vi "Gaussian surface graph.vi"(5 "output cluster":T1, 9 "plot number (1)":i32=2, 10 "X":dbl[](array[numeric]), 11 "Y":dbl[](array[numeric])) -> (0 "error out":errorcluster)   [LabVIEW 2023]
doc: "Generate Gaussian surface graph."
uses:
  <vilib>/Native 3D Graph/xcontrol/3DPC_SurfacePlot.xctl
  <vilib>/Native 3D Graph/classes/Base Datatype.lvclass
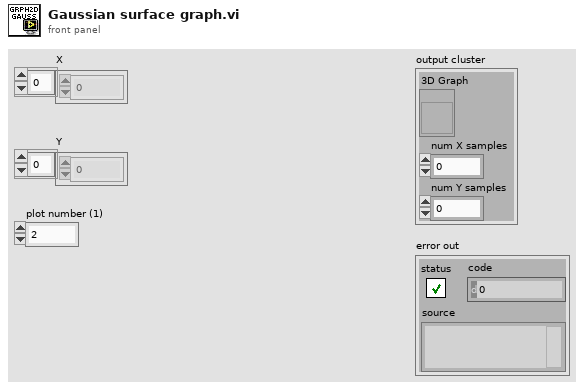
[diagram p1: front panel]
types:
  T1 = cluster{"3D Graph":refnum<vi>, "num X samples":i32, "num Y samples":i32}
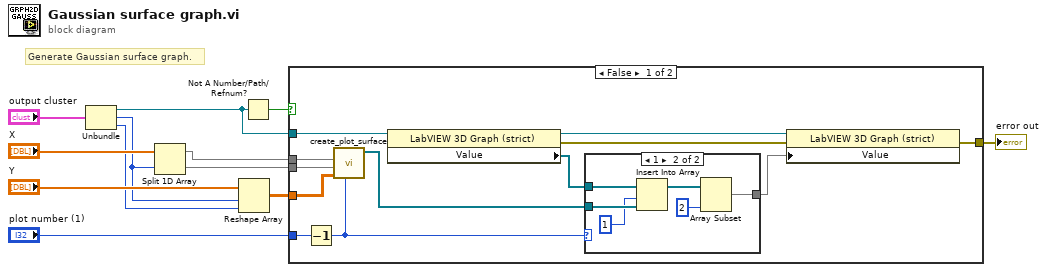
[diagram p0: block diagram]
diagram:
  # "Generate Gaussian surface graph."
  n1 = Unbundle("output cluster") -> ("3D Graph"=w2:refnum<vi>, "num X samples"=w5:i32, "num Y samples"=w4:i32)
  n2 = Split 1D Array(array="X", index=w5) -> (first subarray=w8:dbl[], second subarray=w7:dbl[])
  n3 = Reshape Array("Y", w5, w4) -> (w11:dbl[][])
  n4 = Not A Number/Path/Refnum?(number/path/refnum=w2) -> (NaN/Path/Refnum?=w12:bool)
  n5 = case shown="False" w12 {
    tunnel: w8 -> [w24 _]
    tunnel: w7 -> [w23 _]
    tunnel: w11 -> [w22 _]
    tunnel: w2 -> [w20 _]
    tunnel: "plot number (1)" -> [w19 _]
    tunnel: [w21 _] -> w3
    frame False {
      n6 = Decrement(x=w19) -> (x-1=w14:i32)
      n7 = call <vilib>:"create_plot_surface.vi"("plot ID"=w14, "z matrix"=w22, "y vector"=w23, "x vector"=w24) -> ("plots out"=w15:refnum<class "Base Datatype.lvclass">[])  [unwired: 1 in, 6 out]
      n8 = property class="LabVIEW 3D Graph (strict)"(reference=w20) -> (reference out=w18:refnum<vi>, error out=w16:errorcluster, "Value"=w13:refnum<class "Base Datatype.lvclass">[])  [unwired: 1 in]
      n9 = case shown="1" w14 {
        tunnel: w15 -> [w25 w30]
        tunnel: [w25 w26] -> w17
        tunnel: w13 -> [_ w31]
        frame Default {
        }
        frame 1 {
          n10 = Insert Into Array(array=w31, index=1, new element=w30) -> (w28:refnum<class "Base Datatype.lvclass">[])
          n11 = Array Subset(array=w28, length=2) -> (w26:refnum<class "Base Datatype.lvclass">[])  [unwired: 1 in]
        }
      }
      n12 = property class="LabVIEW 3D Graph (strict)"(reference=w18, error in=w16, "Value"=w17) -> (error out=w21:errorcluster)  [unwired: 1 out]
    }
    frame True {
    }
  }
  "error out" <- w3
